vi "RampTrigger.vi"(5 "Curr B":dbl, 7 "Curr T":dbl, 8 "error in":errorcluster, 9 "dt Trig":bool, 10 "VNACluster In":T1={"Value"=0.0, "GUI Data Cluster"={"S11"=FALSE, "S21"=FALSE, "S12"=FALSE, "S22"=FALSE, "S11Meas"=enum."Log-magnitude (dB)", "S21Meas"=enum."Log-magnitude (dB)", "S12Meas"=enum."Log-magnitude (dB)", "S22Meas"=enum."Log-magnitude (dB)"}, "Timing"={"Last Operation"=0.0, "Stop @ T/B"=FALSE, "Last Temp"=0.0, "Last Mag"=0.0, "Ramp Param"={"End T (K)"=0.0, "Delta T (K)"=0.0, "End B (T)"=0.0, "Delta B (T)"=0.0}, "LastOp?"=FALSE, "FirstOp?"=FALSE}, "Measurements"=[], "Hardware"={"VNA TCP Con"=refnum, "VNA TCP Port"=5025, "Global T VAR"="", "Global B VAR"=""}, "Operation"={"Operation Mode"=enum."Logging", "Log Folder"=path "", "Measure Mode"=enum."Deltat"}}, 11 "Ramp Dir":bool) -> (0 "error out":errorcluster, 2 "VNACluster Out":T1={"Value"=0.0, "GUI Data Cluster"={"S11"=FALSE, "S21"=FALSE, "S12"=FALSE, "S22"=FALSE, "S11Meas"=enum."Log-magnitude (dB)", "S21Meas"=enum."Log-magnitude (dB)", "S12Meas"=enum."Log-magnitude (dB)", "S22Meas"=enum."Log-magnitude (dB)"}, "Timing"={"Last Operation"=0.0, "Stop @ T/B"=FALSE, "Last Temp"=0.0, "Last Mag"=0.0, "Ramp Param"={"End T (K)"=0.0, "Delta T (K)"=0.0, "End B (T)"=0.0, "Delta B (T)"=0.0}, "LastOp?"=FALSE, "FirstOp?"=FALSE}, "Measurements"=[], "Hardware"={"VNA TCP Con"=refnum, "VNA TCP Port"=5025, "Global T VAR"="", "Global B VAR"=""}, "Operation"={"Operation Mode"=enum."Logging", "Log Folder"=path "", "Measure Mode"=enum."Deltat"}}, 4 "Trigger":bool)   [LabVIEW 2021]
uses:
  Data_Cluster.ctl
  Measurement_Cluster.ctl
  Mode_Enum.ctl
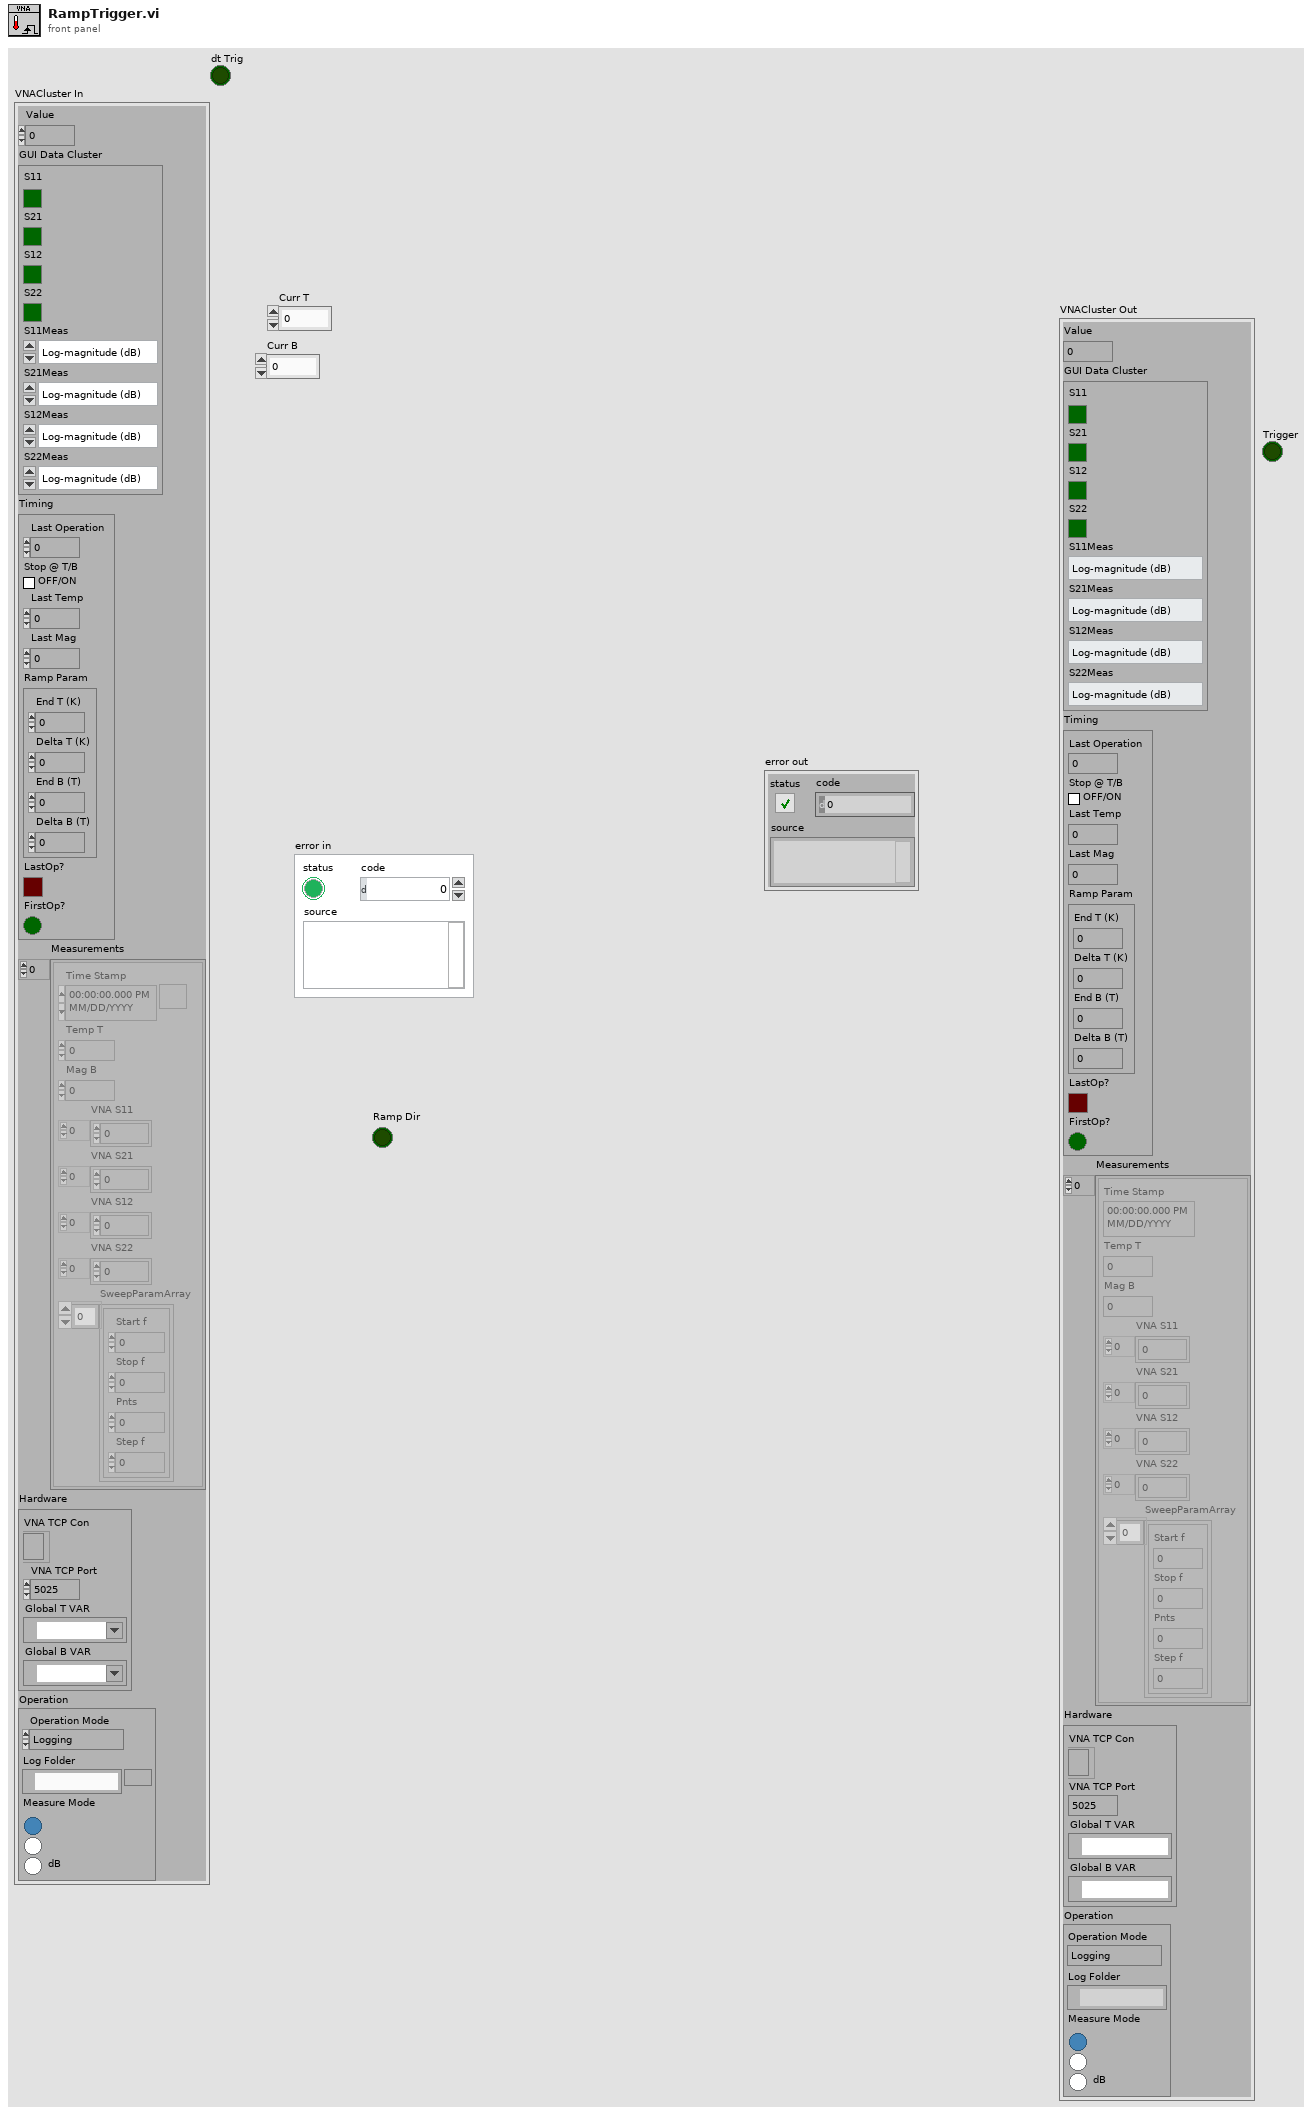
[diagram p1: front panel]
types:
  T1 = typedef "Data_Cluster.ctl" = cluster{"Value":dbl, "GUI Data Cluster":cluster{"S11":bool, "S21":bool, "S12":bool, "S22":bool, "S11Meas":enum16{"Log-magnitude (dB)", "Linear magnitude", "Phase (deg)", "Time Domain", "Real", "Imaginary", "Group Delay", "Polarlinear"}, "S21Meas":enum16{"Log-magnitude (dB)", "Linear magnitude", "Phase (deg)", "Time Domain", "Real", "Imaginary", "Group Delay", "Polarlinear"}, "S12Meas":enum16{"Log-magnitude (dB)", "Linear magnitude", "Phase (deg)", "Time Domain", "Real", "Imaginary", "Group Delay", "Polarlinear"}, "S22Meas":enum16{"Log-magnitude (dB)", "Linear magnitude", "Phase (deg)", "Time Domain", "Real", "Imaginary", "Group Delay", "Polarlinear"}}, "Timing":cluster{"Last Operation":dbl, "Stop @ T/B":bool, "Last Temp":dbl, "Last Mag":dbl, "Ramp Param":cluster{"End T (K)":dbl, "Delta T (K)":dbl, "End B (T)":dbl, "Delta B (T)":dbl}, "LastOp?":bool, "FirstOp?":bool}, "Measurements":T2[], "Hardware":cluster{"VNA TCP Con":refnum<k5>, "VNA TCP Port":i32, "Global T VAR":refnum<k21>, "Global B VAR":refnum<k21>}, "Operation":cluster{"Operation Mode":T3, "Log Folder":path, "Measure Mode":enum32{"Deltat", "DeltaT", "dB"}}}
  T2 = typedef "Measurement_Cluster.ctl" = cluster{"Time Stamp":timestamp, "Temp T":dbl, "Mag B":dbl, "VNA S11":dbl[], "VNA S21":dbl[], "VNA S12":dbl[], "VNA S22":dbl[], "SweepParamArray":cluster{"Start f":dbl, "Stop f":dbl, "Pnts":i32, "Step f":dbl}[]}
  T3 = typedef "Mode_Enum.ctl" = enum16{"Logging", "Idle-Off", "Idle"}
  T4 = cluster{"End T (K)":dbl, "Delta T (K)":dbl, "End B (T)":dbl, "Delta B (T)":dbl}
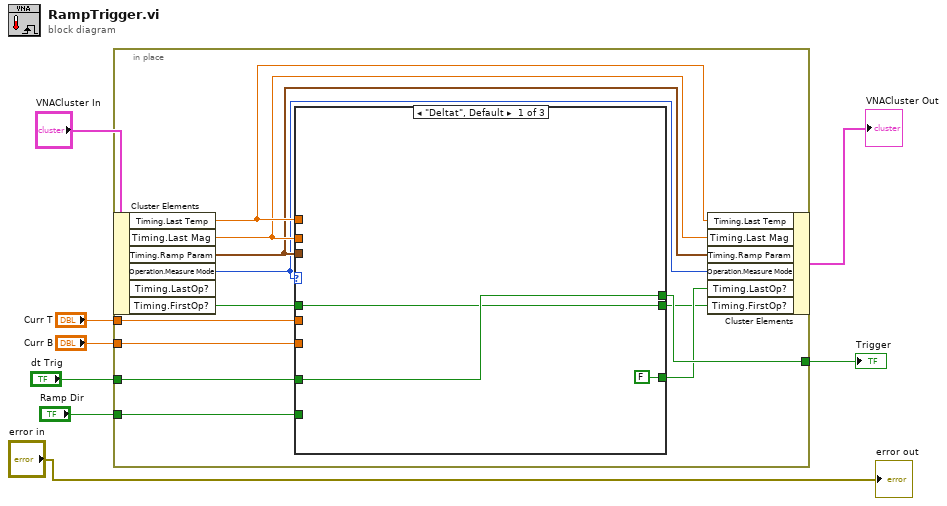
[diagram p0: block diagram]
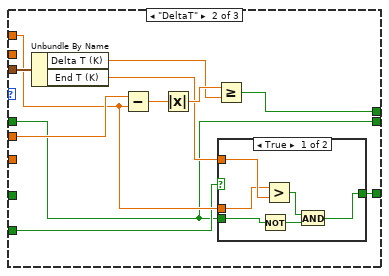
[diagram p2: hidden frame]
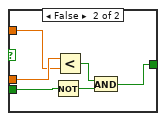
[diagram p3: hidden frame]
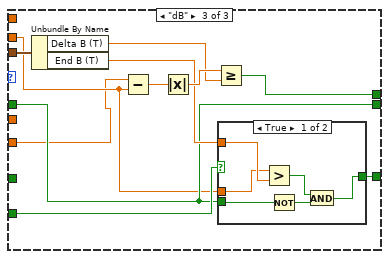
[diagram p4: hidden frame]
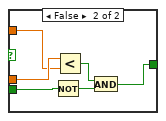
[diagram p5: hidden frame]
diagram:
  n1 = in-place {
    in-place-border: "dt Trig" -> [w20]
    in-place-border: [w19] -> w4
    in-place-border: "Curr T" -> [w14]
    in-place-border: "Curr B" -> [w13]
    in-place-border: "Ramp Dir" -> [w11]
    n2 = in-place-cluster #1("VNACluster In") -> ("Timing.Last Temp"=w18:dbl, "Timing.Last Mag"=w17:dbl, "Timing.Ramp Param"=w16:T4, "Operation.Measure Mode"=w15:enum32{"Deltat", "DeltaT", "dB"}, "Timing.FirstOp?"=w10:bool)  [unwired: 1 out]
    n3 = case shown="\"Deltat\", Default" w15 {
      tunnel: [w23 w31 w54] -> w19
      tunnel: w20 -> [w23 _ _]
      tunnel: w18 -> [_ w26 _]
      tunnel: w17 -> [_ _ w48]
      tunnel: w16 -> [_ w34 w57]
      tunnel: w14 -> [_ w27 _]
      tunnel: w13 -> [_ _ w47]
      tunnel: [FALSE w28 w51] -> w12
      tunnel: w11 -> [_ w25 w50]
      tunnel: w10 -> [w21 w24 w49]
      tunnel: [w21 w24 w49] -> w9
      frame "Deltat", Default {
      }
      frame "DeltaT" {
        n4 = Unbundle By Name(w34) -> ("Delta T (K)"=w32:dbl, "End T (K)"=w29:dbl)
        n5 = Subtract(x=w27, y=w26) -> (x-y=w30:dbl)
        n6 = Absolute Value(x=w30) -> (abs(x)=w33:dbl)
        n7 = Greater Or Equal?(x=w33, y=w32) -> (x >= y?=w31:bool)
        n8 = case shown="True" w25 {
          tunnel: w29 -> [w40 w45]
          tunnel: w26 -> [w39 w46]
          tunnel: [w37 w44] -> w28
          tunnel: w24 -> [w35 w41]
          frame True {
            n9 = Not(x=w35) -> (.not. x?=w36:bool)
            n10 = Greater?(x=w39, y=w40) -> (0:w38:bool)
            n11 = And(x=w38, y=w36) -> (x .and. y?=w37:bool)
          }
          frame False {
            n12 = Not(x=w41) -> (.not. x?=w42:bool)
            n13 = Less?(x=w46, y=w45) -> (x < y?=w43:bool)
            n14 = And(x=w43, y=w42) -> (x .and. y?=w44:bool)
          }
        }
      }
      frame "dB" {
        n15 = Unbundle By Name(w57) -> ("Delta B (T)"=w55:dbl, "End B (T)"=w52:dbl)
        n16 = Subtract(x=w47, y=w48) -> (x-y=w53:dbl)
        n17 = Absolute Value(x=w53) -> (abs(x)=w56:dbl)
        n18 = Greater Or Equal?(x=w56, y=w55) -> (x >= y?=w54:bool)
        n19 = case shown="True" w50 {
          tunnel: w52 -> [w63 w68]
          tunnel: w48 -> [w62 w69]
          tunnel: [w61 w67] -> w51
          tunnel: w49 -> [w58 w64]
          frame True {
            n20 = Greater?(x=w62, y=w63) -> (0:w60:bool)
            n21 = Not(x=w58) -> (.not. x?=w59:bool)
            n22 = And(x=w60, y=w59) -> (x .and. y?=w61:bool)
          }
          frame False {
            n23 = Not(x=w64) -> (.not. x?=w65:bool)
            n24 = Less?(x=w69, y=w68) -> (x < y?=w66:bool)
            n25 = And(x=w66, y=w65) -> (x .and. y?=w67:bool)
          }
        }
      }
    }
    n26 = in-place-cluster #1("Timing.Last Temp"=w18, "Timing.Last Mag"=w17, "Timing.Ramp Param"=w16, "Operation.Measure Mode"=w15, "Timing.LastOp?"=w12, "Timing.FirstOp?"=w9) -> (→"VNACluster Out":T1)
  }
  "Trigger" <- w4
  "error out" <- "error in"
